vi "Close Client.vi"(8 "error in (no error)":errorcluster, 11 "Client Ref":T1) -> (0 "error out":errorcluster)   [LabVIEW 2019, in "Template Client.lvlib" / "gprc-lvsupport.lvlib"]
uses:
  gprc-lvsupport.lvlib
  Server API/typeDefs/grpcId.ctl
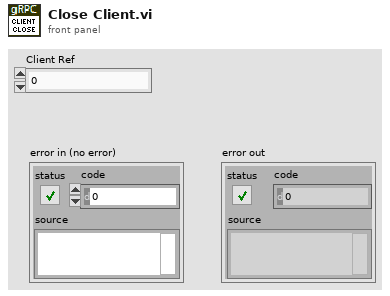
[diagram p1: front panel]
types:
  T1 = typedef "Template Client.lvlib/gprc-lvsupport.lvlib/grpcId.ctl" = u64
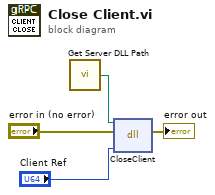
[diagram p0: block diagram]
diagram:
  n1 = call "Get Server DLL Path.vi"() -> ("Server dll path"=w3:path)
  n2 = dll-call lib="?" fn="CloseClient"(path in=w3, error in="error in (no error)", "clientId"="Client Ref") -> (error out=→"error out":errorcluster)  [unwired: 3 in, 1 out]
